vi "Actor Core.vi"(8 "error in":errorcluster, 11 "OneButtonDialogBox In":refnum<class "TwoButtonDialogBox.lvclass">) -> (0 "error out":errorcluster, 3 "Actor out":refnum<class "Actor.lvclass">)   [LabVIEW 2015, in "TwoButtonDialogBox.lvlib" / "TwoButtonDialogBox.lvclass"]
doc: "(<B>Filename</B>: Actor Framework.lvlib:Actor.lvclass:Actor Core.vi)\n\nReceives messages to the actor, reacts to them, and initiates any error handling that may shut the actor down.\n\nDescendant classes may override this VI to append parallel tasks for the actor to complete while it handles messages. Overrides use the Call Parent Method node."
uses:
  TwoButtonDialogBox.lvclass
  <vilib>/ActorFramework/Actor/Actor.lvclass
  <vilib>/ActorFramework/Actor/Actor.lvclass/Actor.ctl
  <vilib>/ActorFramework/Message Enqueuer/Message Enqueuer.lvclass/Message Enqueuer.ctl
  TwoButtonDialogBox.lvclass/TwoButtonDialogBox.ctl
  <vilib>/ActorFramework/Message Enqueuer/Init from Existing Queue.vi
  IDialogBox/IDialogBox/IDialogBox.lvclass
  <vilib>/ActorFramework/Message Enqueuer/Message Enqueuer.lvclass
  AutoRegistration/ActorAutoRegistration/ActorAutoRegistration.lvclass
panel:
  in  "False":bool
  out "Message Text":string
  in  "True":bool
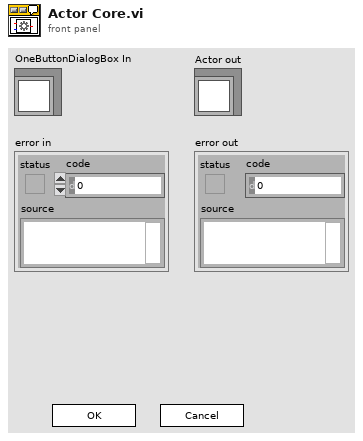
[diagram p1: front panel]
types:
  T1 = enum32{"Invalid", "Default", "Floating", "Floating/Auto-Hide", "Modal"}
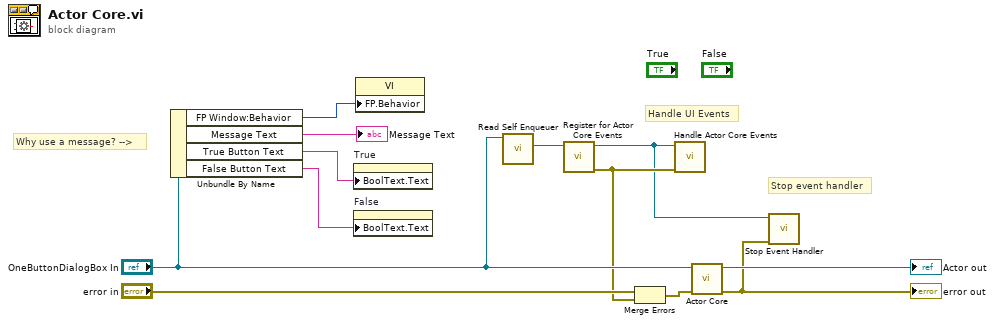
[diagram p0: block diagram]
diagram:
  # "Stop event handler"
  # "Handle UI Events"
  # "Why use a message? -->"
  n1 = Unbundle By Name("OneButtonDialogBox In") -> ("FP Window:Behavior"=w1:T1, "Message Text"=→"Message Text":string, "True Button Text"=w10:string, "False Button Text"=w9:string)
  n2 = property on="True" class="Bool"("BoolText.Text"=w10) -> ()  [unwired: 2 in, 2 out]
  n3 = property on="False" class="Bool"("BoolText.Text"=w9) -> ()  [unwired: 2 in, 2 out]
  n4 = property class="VI"("FP.Behavior"=w1) -> ()  [unwired: 2 in, 2 out]
  n5 = call <vilib>:"Read Self Enqueuer.vi"("Actor"="OneButtonDialogBox In") -> ("Self Enqueuer"=w8:refnum<class "Message Enqueuer.lvclass">)  [unwired: 10 in]
  n6 = call "Register for Actor Core Events.vi"("Actor Enqueuer"=w8) -> ("error out"=w3:errorcluster, "ActorAutoRegistration Out"=w2:refnum<class "ActorAutoRegistration.lvclass">)  [unwired: 9 in]
  n7 = Merge Errors("error in", w3) -> (w5:errorcluster)
  n8 = call-dynamic "Handle Actor Core Events.vi"("error in (no error)"=w3, "ActorAutoRegistration in"=w2) -> ()  [unwired: 9 in, 1 out]
  n9 = call-parent "Actor Core.vi"("error in"=w5, "IViewable In"="OneButtonDialogBox In") -> ("error out"=w4:errorcluster, "Actor out"=→"Actor out":refnum<class "Actor.lvclass">)  [unwired: 8 in]
  "error out" <- w4
  n10 = call-dynamic "Stop Event Handler.vi"("error in (no error)"=w4, "ActorAutoRegistration in"=w2) -> ()  [unwired: 9 in, 1 out]
